vi "Main.vi"() -> ()   [LabVIEW 2014]
doc: "The boiler controller allows a user to start and shut down a boiler.\n\nUse the Reset, Start, and Light Pilot controls to sequentially start the boiler. \nUse the Fuel Control Valve to change the flow of fuel into the boiler. \nUse the Stop Boiler button to shut down the boiler. \nTo shut down the system or in the event of an emergency, use the Emergency Stop button to close the application completely."
uses:
  controls/MHL Data.ctl
  controls/MHL UI Data.ctl
  controls/MHL Status.ctl
  controls/MHL References.ctl
  controls/MHL Configuration.ctl
  support/Boiler System Globals.vi
  <vilib>/Utility/error.llb/Error Cluster From Error Code.vi
  <vilib>/ErrorRing/Error Ring.xnode
  support/Message Queue/Message Queue.lvlib
  support/User Event - Stop/User Event - Stop.lvlib
  Controller/Controller.lvlib
  Boiler/Boiler.lvlib
panel:
  in  "Fuel Control Valve":u32(slide) min=10 max=75 scale=10.0..75.0
  in  "Stop Boiler":bool
  in  "Light Pilot":bool
  out "Forced Draft Fan":bool
  out "Pilot":bool
  out "Pilot Gas Valve":bool
  out "Primary Fan":bool
  out "Status":string
  in  "Start":bool
  in  "Reset":bool
  in  "Emergency Stop":bool
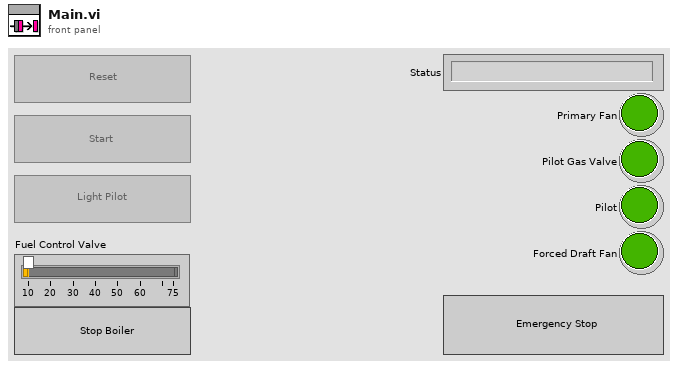
[diagram p1: front panel]
types:
  T1 = typedef "MHL Data.ctl" = cluster{"MHL User Interface Data":T2, "MHL References":T4, "MHL Configuration":T5}
  T2 = typedef "MHL UI Data.ctl" = cluster{"Status":string, "Fuel Control Valve":u32, "Primary Fan":bool, "Pilot Gas Valve":bool, "Pilot":bool, "Forced Draft Fan":bool, "MHL Status":T3}
  T3 = typedef "MHL Status.ctl" = enum16{"Lockout", "Ready", "Pre-Purge", "Pre-Purge Complete", "Pilot On", "Boiler Running", "Shutdown", "Purge"}
  T4 = typedef "MHL References.ctl" = cluster{"Reset Ref":refnum<vi>, "Start Ref":refnum<vi>, "Light Pilot Ref":refnum<vi>, "Stop Boiler Ref":refnum<vi>, "Fuel Control Valve Ref":refnum<vi>}
  T5 = typedef "MHL Configuration.ctl" = cluster{"Fuel Control Valve Maximum":dbl, "Fuel Control Valve Minimum":dbl}
  T6 = typedef "Configuration Data.ctl" = cluster{"MHL Configuration":T5, "Controller Configuration":T7, "Boiler Configuration":T8}
  T7 = typedef "Controller.lvlib/Controller Configuration.ctl" = cluster{"Purge Time":u32, "Flame Threshold":u32}
  T8 = typedef "Boiler.lvlib/Boiler Configuration.ctl" = cluster{"Pilot Increment (ms)":u32, "Pilot Decrement (ms)":u32}
  T9 = typedef "Notifiers.ctl" = cluster{"Handshake":refnum<notifier>, "Flame Level":refnum<notifier>, "Controller Exit":refnum<notifier>, "Boiler Exit":refnum<notifier>}
  T10 = typedef "Message Queue.lvlib/All Message Queues.ctl" = cluster{"MHL":refnum<queue>, "Boiler Controller":refnum<queue>, "Boiler":refnum<queue>}
  T11 = enum16{"open", "replace", "create", "open or create", "replace or create", "replace or create with confirmation"}
  T12 = enum32{"invalid app kind", "Development System", "Run Time System", "Student Edition", "Embedded LabVIEW", "Evaluation", "Custom"}
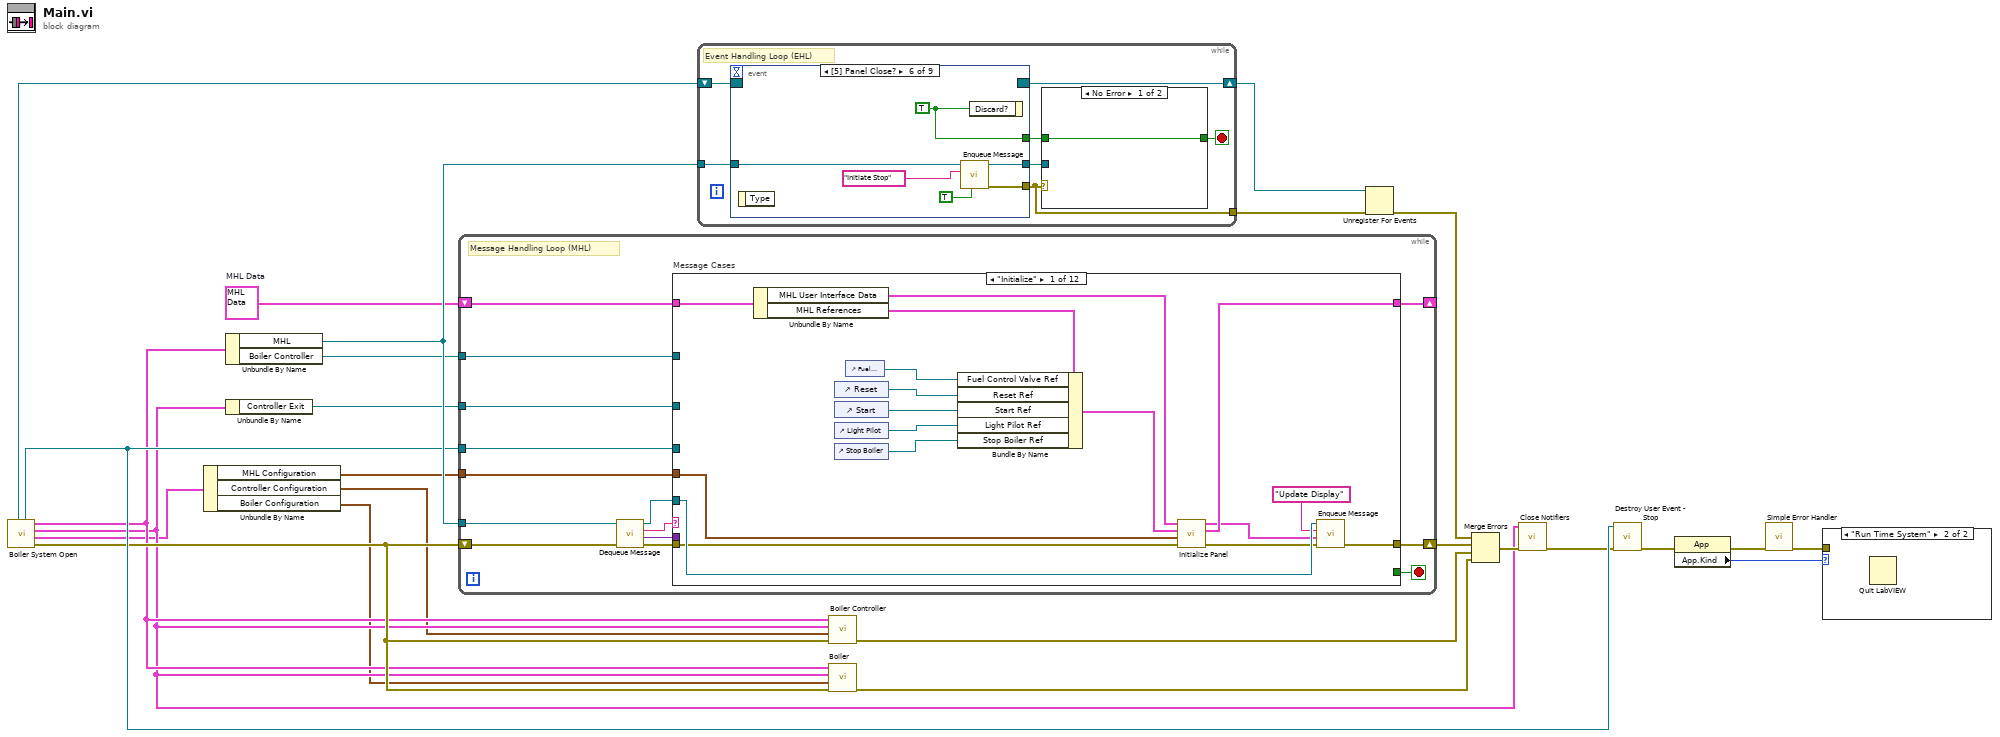
[diagram p0: block diagram]
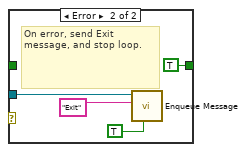
[diagram p3: hidden frame]
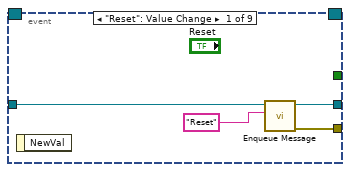
[diagram p4: hidden frame]
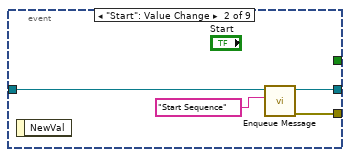
[diagram p5: hidden frame]
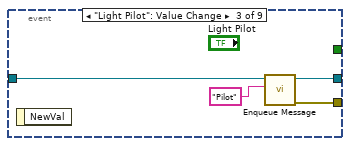
[diagram p6: hidden frame]
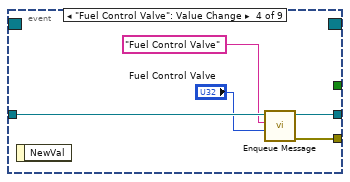
[diagram p7: hidden frame]
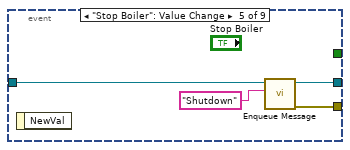
[diagram p8: hidden frame]
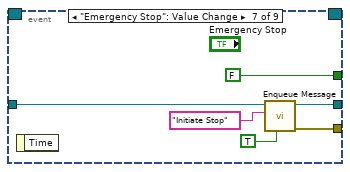
[diagram p9: hidden frame]
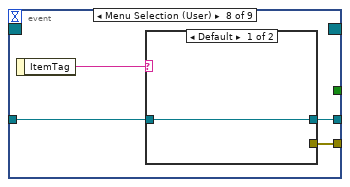
[diagram p10: hidden frame]
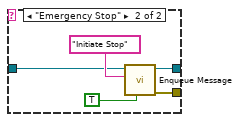
[diagram p11: hidden frame]
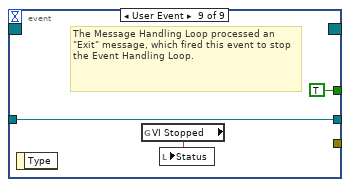
[diagram p12: hidden frame]
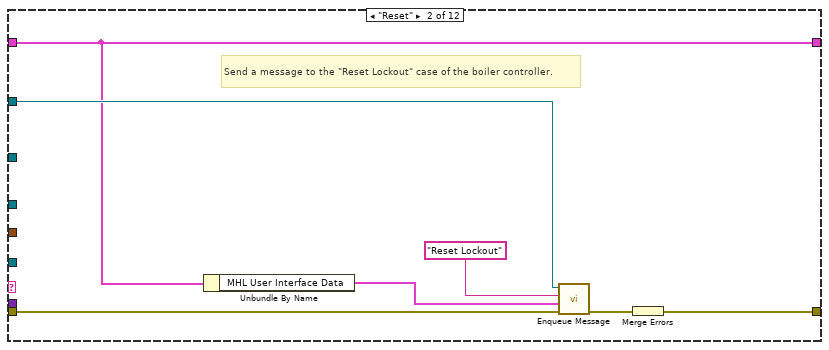
[diagram p13: hidden frame]
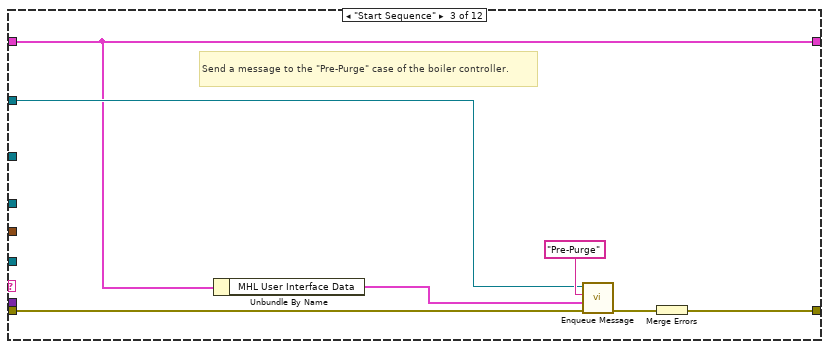
[diagram p14: hidden frame]
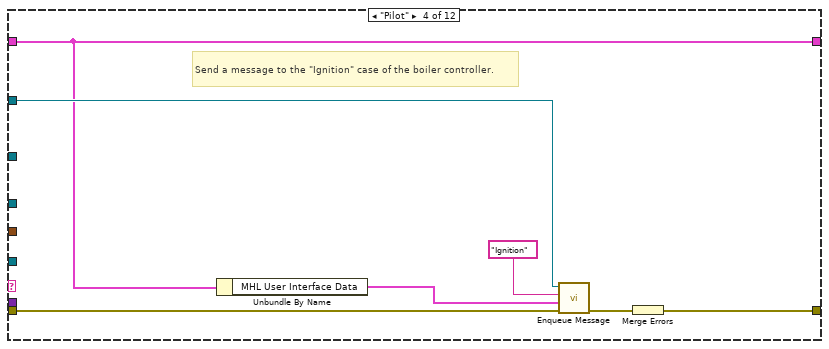
[diagram p15: hidden frame]
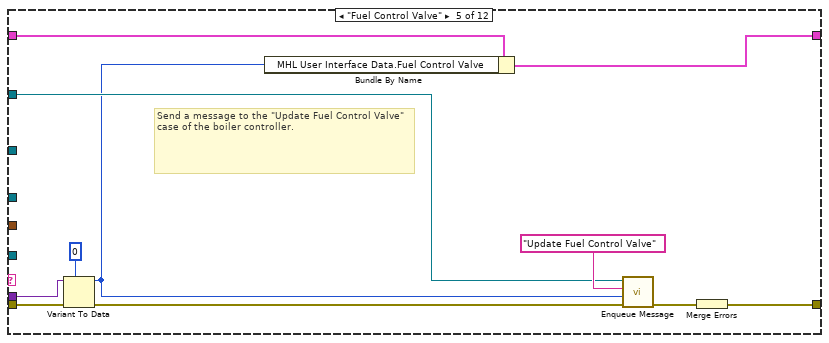
[diagram p16: hidden frame]
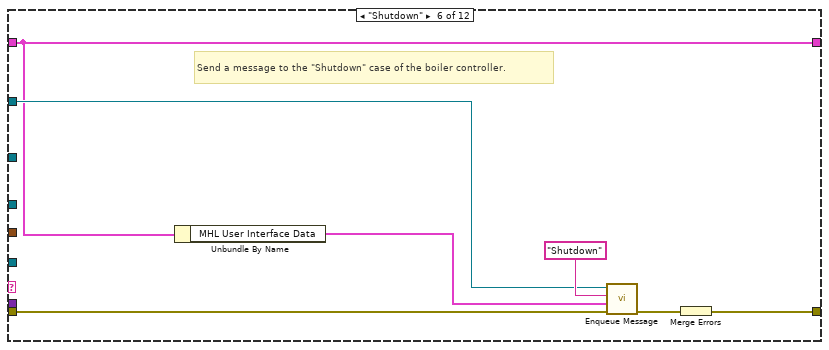
[diagram p17: hidden frame]
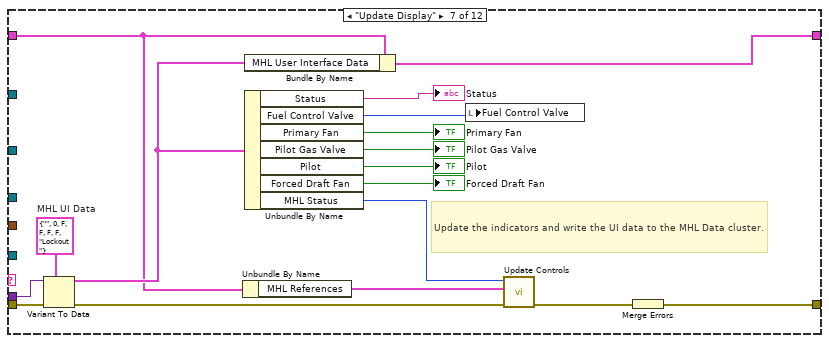
[diagram p18: hidden frame]
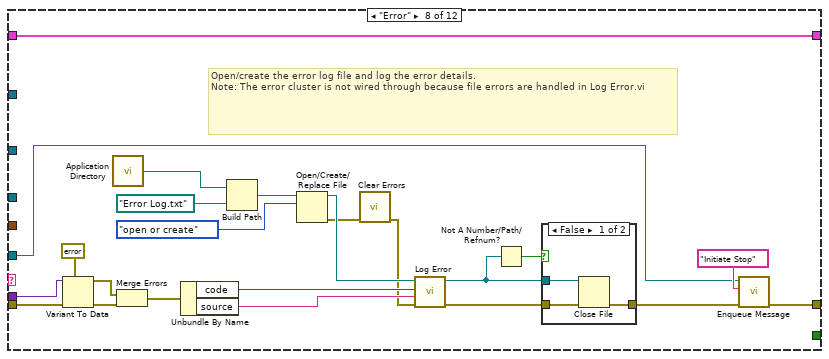
[diagram p19: hidden frame]
diagram:
  w19 = T1 {"MHL User Interface Data"={"Status"="", "Fuel Control Valve"=0, "Primary Fan"=FALSE, "Pilot Gas Valve"=FALSE, "Pilot"=FALSE, "Forced Draft Fan"=FALSE, "MHL Status"=enum."Lockout"}, "MHL References"={"Reset Ref"=refnum, "Start Ref"=refnum, "Light Pilot Ref"=refnum, "Stop Boiler Ref"=refnum, "Fuel Control Valve Ref"=refnum}, "MHL Configuration"={"Fuel Control Valve Maximum"=0.0, "Fuel Control Valve Minimum"=0.0}}  # MHL Data
  n1 = call "Boiler System Open.vi"() -> ("error out"=w10:errorcluster, "Configuration Data"=w4:T6, "Notifiers"=w5:T9, "Message Queues"=w9:T10, "User Event - Stop"=w12:refnum<user-event>, "Stop Event Registration Refnum"=w13:refnum<event-registration>)  [unwired: 6 in]
  n2 = Unbundle By Name(w4) -> ("MHL Configuration"=w3:T5, "Controller Configuration"=w2:T7, "Boiler Configuration"=w1:T8)
  n3 = Unbundle By Name(w9) -> ("MHL"=w24:refnum<queue>, "Boiler Controller"=w17:refnum<queue>)
  n4 = Unbundle By Name(w5) -> ("Controller Exit"=w11:refnum<notifier>)
  n5 = while {
    tunnel: w24 -> [w29]
    shift-right: [w38] -> _
    shift-left: w19 -> [w39]
    tunnel: w12 -> [w35]
    shift-right: [w36] -> w25
    shift-left: w10 -> [w34]
    tunnel: w17 -> [w28]
    tunnel: w11 -> [w27]
    tunnel: w3 -> [w26]
    stop <- w37 stop-if-true
    # "Message Handling Loop (MHL)"
    n6 = call "Dequeue Message.vi"("error in (no error)"=w34, "Message Queue"=w29) -> ("error out"=w33:errorcluster, "Message Data"=w31:variant, "Message"=w32:string, "dup Message Queue"=w30:refnum<queue>)  [unwired: 6 in]
    n7 = case "Message Cases" shown="\"Initialize\"" w32 {
      selector: w32 -> [_ _ _ _ _ _ _ _ _ _ _ w173]
      tunnel: w30 -> [w49 _ _ _ _ _ _ w121 w142 w149 w171 _]
      tunnel: w33 -> [w43 w62 w69 w76 w84 w94 w111 w119 w147 w151 w164 _]
      tunnel: [w50 w63 w70 w77 w88 w95 w112 w117 w144 w150 w167 w172] -> w36
      tunnel: w39 -> [w51 w58 w65 w72 w80 w90 w97 w135 w146 w155 w170 w174]
      tunnel: [w41 w58 w65 w72 w79 w90 w101 w135 w146 w155 w170 w174] -> w38
      tunnel: [_ _ _ _ _ _ _ _ _ _ TRUE _] -> w37
      tunnel: w31 -> [_ _ _ _ w82 _ w110 w118 _ _ _ _]
      tunnel: w35 -> [_ _ _ _ _ _ _ _ _ _ w166 _]
      tunnel: w28 -> [_ w59 w66 w73 w85 w91 _ _ w143 _ _ _]
      tunnel: w27 -> [_ _ _ _ _ _ _ _ _ w148 _ _]
      tunnel: w26 -> [w47 _ _ _ _ _ _ _ _ _ _ _]
      frame "Initialize" {
        n8 = Unbundle By Name(w51) -> ("MHL User Interface Data"=w44:T2, "MHL References"=w45:T4)
        n9 = control-ref of="Reset"() -> (w53:refnum<vi>)
        n10 = control-ref of="Start"() -> (w54:refnum<vi>)
        n11 = control-ref of="Light Pilot"() -> (w55:refnum<vi>)
        n12 = control-ref of="Stop Boiler"() -> (w56:refnum<vi>)
        n13 = control-ref of="Fuel Control Valve"() -> (w52:refnum<vi>)
        n14 = Bundle By Name(cluster=w45, "Fuel Control Valve Ref"=w52, "Reset Ref"=w53, "Start Ref"=w54, "Light Pilot Ref"=w55, "Stop Boiler Ref"=w56) -> (w46:T4)
        n15 = call "Initialize Panel.vi"("error in"=w43, "MHL Configuration"=w47, "MHL References"=w46, "MHL UI Data in"=w44) -> ("error out"=w42:errorcluster, "MHL Data out"=w41:T1, "MHL UI Data out"=w40:T2)  [unwired: 5 in]
        n16 = call "Enqueue Message.vi"("error in (no error)"=w42, "Message Data"=w40, "Message"="Update Display", "Message Queue"=w49) -> ("error out"=w50:errorcluster)  [unwired: 6 in, 1 out]
      }
      frame "Reset" {
        # "Send a message to the \"Reset Lockout\" case of the boiler controller."
        n17 = Unbundle By Name(w58) -> ("MHL User Interface Data"=w57:T2)
        n18 = call "Enqueue Message.vi"("error in (no error)"=w62, "Message Data"=w57, "Message"="Reset Lockout", "Message Queue"=w59) -> ("error out"=w61:errorcluster)  [unwired: 6 in, 1 out]
        n19 = Merge Errors(w61) -> (w63:errorcluster)
      }
      frame "Start Sequence" {
        # "Send a message to the \"Pre-Purge\" case of the boiler controller."
        n20 = Unbundle By Name(w65) -> ("MHL User Interface Data"=w64:T2)
        n21 = call "Enqueue Message.vi"("error in (no error)"=w69, "Message Data"=w64, "Message"="Pre-Purge", "Message Queue"=w66) -> ("error out"=w68:errorcluster)  [unwired: 6 in, 1 out]
        n22 = Merge Errors(w68) -> (w70:errorcluster)
      }
      frame "Pilot" {
        # "Send a message to the \"Ignition\" case of the boiler controller."
        n23 = Unbundle By Name(w72) -> ("MHL User Interface Data"=w71:T2)
        n24 = call "Enqueue Message.vi"("error in (no error)"=w76, "Message Data"=w71, "Message"="Ignition", "Message Queue"=w73) -> ("error out"=w75:errorcluster)  [unwired: 6 in, 1 out]
        n25 = Merge Errors(w75) -> (w77:errorcluster)
      }
      frame "Fuel Control Valve" {
        # "Send a message to the \"Update Fuel Control Valve\" case of the boiler controller."
        n26 = Variant To Data(error in=w84, type=u32 0 ("Fuel Control Valve"), Variant=w82) -> (data=w78:u32, error out=w83:errorcluster)
        n27 = Bundle By Name(cluster=w80, "MHL User Interface Data.Fuel Control Valve"=w78) -> (w79:T1)
        n28 = call "Enqueue Message.vi"("error in (no error)"=w83, "Message Data"=w78, "Message"="Update Fuel Control Valve", "Message Queue"=w85) -> ("error out"=w87:errorcluster)  [unwired: 6 in, 1 out]
        n29 = Merge Errors(w87) -> (w88:errorcluster)
      }
      frame "Shutdown" {
        # "Send a message to the \"Shutdown\" case of the boiler controller."
        n30 = Unbundle By Name(w90) -> ("MHL User Interface Data"=w89:T2)
        n31 = call "Enqueue Message.vi"("error in (no error)"=w94, "Message Data"=w89, "Message"="Shutdown", "Message Queue"=w91) -> ("error out"=w93:errorcluster)  [unwired: 6 in, 1 out]
        n32 = Merge Errors(w93) -> (w95:errorcluster)
      }
      frame "Update Display" {
        w109 = T2 {"Status"="", "Fuel Control Valve"=0, "Primary Fan"=FALSE, "Pilot Gas Valve"=FALSE, "Pilot"=FALSE, "Forced Draft Fan"=FALSE, "MHL Status"=enum."Lockout"}  # MHL UI Data
        # "Update the indicators and write the UI data to the MHL Data cluster."
        n33 = Variant To Data(error in=w111, type=w109, Variant=w110) -> (data=w102:T2, error out=w100:errorcluster)
        n34 = Unbundle By Name(w97) -> ("MHL References"=w96:T4)
        n35 = Bundle By Name(cluster=w97, "MHL User Interface Data"=w102) -> (w101:T1)
        n36 = Unbundle By Name(w102) -> ("Status"=→"Status":string, "Fuel Control Valve"=w107:u32, "Primary Fan"=→"Primary Fan":bool, "Pilot Gas Valve"=→"Pilot Gas Valve":bool, "Pilot"=→"Pilot":bool, "Forced Draft Fan"=→"Forced Draft Fan":bool, "MHL Status"=w98:T3)
        n37 = local write "Fuel Control Valve"(w107) -> ()
        n38 = call "Update Controls.vi"("error in"=w100, "MHL References"=w96, "MHL Status"=w98) -> ("error out"=w99:errorcluster)  [unwired: 8 in]
        n39 = Merge Errors(w99) -> (w112:errorcluster)
      }
      frame "Error" {
        # "Open/create the error log file and log the error details.\nNote: The error cluster is not wired through because file errors are handled in Log Error.vi"
        n40 = Variant To Data(error in=w119, type=errorcluster {"status"=FALSE, "code"=0, "source"=""} ("error out"), Variant=w118) -> (data=w131:errorcluster, error out=w132:errorcluster)
        n41 = call <vilib>:"Application Directory.vi"() -> ("Application Directory"=w129:path)
        n42 = Merge Errors(w131, w132) -> (w130:errorcluster)
        n43 = Unbundle By Name(w130) -> ("code"=w124:i32, "source"=w123:string)
        n44 = Build Path(base path=w129, name or relative path=path "Error Log.txt") -> (appended path=w128:path)
        n45 = Open/Create/Replace File(file path (use dialog)=w128, operation (0:open)=T11."open or create") -> (refnum out=w126:refnum<file>, error out=w114:errorcluster)  [unwired: 4 in, 1 out]
        n46 = call <vilib>:"Clear Errors.vi"("error in (no error)"=w114) -> ("error out"=w113:errorcluster)  [unwired: 5 in, 1 out]
        n47 = call "Log Error.vi"("error in"=w113, "Source"=w123, "Code"=w124, "Error Log Refnum In"=w126) -> ("error out"=w125:errorcluster, "Error Log Refnum Out"=w116:refnum<file>)  [unwired: 6 in]
        n48 = Not A Number/Path/Refnum?(number/path/refnum=w116) -> (NaN/Path/Refnum?=w115:bool)
        n49 = case shown="False" w115 {
          tunnel: w125 -> [w138 w139]
          tunnel: w116 -> [w137 _]
          tunnel: [w136 w139] -> w122
          frame False {
            n50 = Close File(refnum=w137, error in=w138) -> (error out=w136:errorcluster)  [unwired: 1 out]
          }
          frame True {
          }
        }
        n51 = call "Enqueue Message.vi"("error in (no error)"=w122, "Message"="Initiate Stop", "Message Queue"=w121) -> ("error out"=w117:errorcluster)  [unwired: 7 in, 1 out]
      }
      frame "Initiate Stop" {
        # "When stopping, first send a message to stop the boiler controller. Then wait for the boiler and boiler controller to exit."
        n52 = call "Enqueue Message.vi"("error in (no error)"=w147, "Message"="Exit", "Message Queue"=w143) -> ("error out"=w145:errorcluster)  [unwired: 7 in, 1 out]
        n53 = call "Enqueue Message.vi"("error in (no error)"=w145, "Message"="Wait on Boiler Exit", "Message Queue"=w142) -> ("error out"=w144:errorcluster)  [unwired: 7 in, 1 out]
      }
      frame "Wait on Boiler Exit" {
        # "Monitor the boiler controller to determine if it has completed its Exit. Wait 10 milliseconds for the boiler controller to respond. \nIf the notification does not occur, then enqueue another Wait on Boiler Exit message.\nIf the notification occurs, then exit the Message Handling Loop."
        n54 = Wait on Notification(notifier=w148, timeout in ms (-1)=10, error in (no error)=w151) -> (timed out?=w153:bool, error out=w152:errorcluster)  [unwired: 1 in, 2 out]
        n55 = case shown="True" w153 {
          tunnel: w152 -> [w159 w163]
          tunnel: w149 -> [w158 w161]
          tunnel: [w156 w162] -> w150
          frame False {
            n56 = call "Enqueue Message.vi"("error in (no error)"=w159, "Message"="Exit", "Message Queue"=w158) -> ("error out"=w156:errorcluster)  [unwired: 7 in, 1 out]
          }
          frame True {
            n57 = call "Enqueue Message.vi"("error in (no error)"=w163, "Message"="Wait on Boiler Exit", "Message Queue"=w161) -> ("error out"=w162:errorcluster)  [unwired: 7 in, 1 out]
          }
        }
      }
      frame "Exit" {
        # "Stop the VI"
        # "Release the message queue reference"
        n58 = call "Fire User Event - Stop.vi"("User Event - Stop"=w166) -> ("error out"=w165:errorcluster)  [unwired: 10 in]
        n59 = Release Queue(queue=w171, error in (no error)=w164) -> (error out=w168:errorcluster)  [unwired: 1 in, 2 out]
        n60 = Merge Errors(w165, w168) -> (w167:errorcluster)
      }
      frame Default {
        # "'Default' case only runs if there is a message that isn't defined in any of the other cases.  Output a programming error."
        n61 = xnode "Error Ring"("parameter 0"=w173) -> ("error out"=w172:errorcluster)
      }
    }
  }
  n62 = while {
    tunnel: w24 -> [w188]
    tunnel: [w184] -> w21
    shift-right: [w182] -> w20
    shift-left: w13 -> [w183]
    stop <- w186 stop-if-true
    # "Event Handling Loop (EHL)"
    n63 = event shown="[5] Panel Close?" {
      selector: w183 -> [_ _ _ _ _ _ _ _ _]
      dyn-events: [_ _ _ _ _ _ _ _ _] -> w182
      timeout: _ -> [_ _ _ _ _ _ _ _ _]
      tunnel: [_ _ _ _ _ w220 FALSE ("Discard?") _ TRUE ("Discard?")] -> w187
      tunnel: w188 -> [w197 w201 w205 w210 w214 w219 w226 w229 w239]
      tunnel: [w196 w199 w203 w208 w212 w218 w225 w227 _] -> w184
      tunnel: [w195 w200 w204 w209 w213 w217 w223 w228 w239] -> w185
      event "Reset": Value Change {
        n64 = event-data() -> ()  [unwired: 1 in, 1 out]
        n65 = call "Enqueue Message.vi"("Message"="Reset", "Message Queue"=w197) -> ("error out"=w196:errorcluster, "dup Message Queue"=w195:refnum<queue>)  [unwired: 8 in]
      }
      event "Start": Value Change {
        n66 = event-data() -> ()  [unwired: 1 in, 1 out]
        n67 = call "Enqueue Message.vi"("Message"="Start Sequence", "Message Queue"=w201) -> ("error out"=w199:errorcluster, "dup Message Queue"=w200:refnum<queue>)  [unwired: 8 in]
      }
      event "Light Pilot": Value Change {
        n68 = event-data() -> ()  [unwired: 1 in, 1 out]
        n69 = call "Enqueue Message.vi"("Message"="Pilot", "Message Queue"=w205) -> ("error out"=w203:errorcluster, "dup Message Queue"=w204:refnum<queue>)  [unwired: 8 in]
      }
      event "Fuel Control Valve": Value Change {
        n70 = event-data() -> ()  [unwired: 1 in, 1 out]
        n71 = call "Enqueue Message.vi"("Message Data"="Fuel Control Valve", "Message"="Fuel Control Valve", "Message Queue"=w210) -> ("error out"=w208:errorcluster, "dup Message Queue"=w209:refnum<queue>)  [unwired: 7 in]
      }
      event "Stop Boiler": Value Change {
        n72 = event-data() -> ()  [unwired: 1 in, 1 out]
        n73 = call "Enqueue Message.vi"("Message"="Shutdown", "Message Queue"=w214) -> ("error out"=w212:errorcluster, "dup Message Queue"=w213:refnum<queue>)  [unwired: 8 in]
      }
      event Panel Close? {
        w220 = TRUE ("Discard?")
        n74 = event-data() -> ()  [unwired: 1 in, 1 out]
        n75 = call "Enqueue Message.vi"("Priority Message? (F)"=TRUE, "Message"="Initiate Stop", "Message Queue"=w219) -> ("error out"=w218:errorcluster, "dup Message Queue"=w217:refnum<queue>)  [unwired: 7 in]
        n76 = event-data("Discard?"=w220) -> ()  [unwired: 1 in, 1 out]
      }
      event "Emergency Stop": Value Change {
        n77 = event-data() -> ()  [unwired: 1 in, 1 out]
        n78 = call "Enqueue Message.vi"("Priority Message? (F)"=TRUE, "Message"="Initiate Stop", "Message Queue"=w226) -> ("error out"=w225:errorcluster, "dup Message Queue"=w223:refnum<queue>)  [unwired: 7 in]
      }
      event Menu Selection (User) {
        n79 = event-data() -> ("ItemTag"=w230:string)  [unwired: 1 in]
        n80 = case shown="Default" w230 {
          tunnel: w229 -> [w231 w234]
          tunnel: [w231 w233] -> w228
          tunnel: [_ w232] -> w227
          frame Default {
          }
          frame "Emergency Stop" {
            n81 = call "Enqueue Message.vi"("Priority Message? (F)"=TRUE, "Message"="Initiate Stop", "Message Queue"=w234) -> ("error out"=w232:errorcluster, "dup Message Queue"=w233:refnum<queue>)  [unwired: 7 in]
          }
        }
      }
      event User Event {
        # "The Message Handling Loop processed an \"Exit\" message, which fired this event to stop the Event Handling Loop."
        n82 = event-data() -> ()  [unwired: 1 in, 1 out]
        n83 = global read "Boiler System Globals.vi" "VI Stopped"() -> (w237:string)
        n84 = local write "Status"(w237) -> ()
      }
    }
    n85 = case shown="No Error" w184 {
      tunnel: [w189 TRUE ("Discard?")] -> w186
      tunnel: w187 -> [w189 _]
      tunnel: w185 -> [_ w192]
      frame No Error {
      }
      frame Error {
        # "On error, send Exit message, and stop loop."
        n86 = call "Enqueue Message.vi"("Priority Message? (F)"=TRUE, "Message"="Exit", "Message Queue"=w192) -> ()  [unwired: 7 in, 2 out]
      }
    }
  }
  n87 = call "Boiler Controller.vi"("error in"=w10, "Controller Configuration"=w2, "Notifiers"=w5, "Message Queues"=w9) -> ("error out"=w18:errorcluster)  [unwired: 7 in]
  n88 = call "Boiler.vi"("error in"=w10, "Boiler Configuration"=w1, "Notifiers"=w5, "Message Queues"=w9) -> ("error out"=w8:errorcluster)  [unwired: 7 in]
  n89 = Unregister For Events(event registration refnum=w20, error in=w21) -> (error out=w22:errorcluster)
  n90 = Merge Errors(w22, w25, w18, w8) -> (w7:errorcluster)
  n91 = call "Close Notifiers.vi"("error in"=w7, "Notifiers"=w5) -> ("error out"=w6:errorcluster)  [unwired: 9 in]
  n92 = call "Destroy User Event - Stop.vi"("error in (no error)"=w6, "User Event - Stop"=w12) -> ("error out"=w23:errorcluster)  [unwired: 9 in]
  n93 = property class="App"(error in=w23) -> (error out=w16:errorcluster, "App.Kind"=w15:T12)  [unwired: 1 in, 1 out]
  n94 = call <vilib>:"Simple Error Handler.vi"("error in (no error)"=w16) -> ("error out"=w14:errorcluster)  [unwired: 4 in, 4 out]
  n95 = case shown="\"Run Time System\"" w15 {
    tunnel: w14 -> [_ _]
    frame Default {
    }
    frame "Run Time System" {
      n96 = Quit LabVIEW() -> ()  [unwired: 1 in]
    }
  }
